vi "Get value by Variant.vi"(8 "error in (no error)":errorcluster, 11 "Numeric Column in":refnum<class "Numeric Column.lvclass">) -> (0 "error out":errorcluster, 2 "Variant":variant, 3 "Numeric Column out":refnum<class "Numeric Column.lvclass">)   [LabVIEW 2020, in "Basic Columns.lvlib" / "Numeric Column.lvclass"]
uses:
  Numeric Column.lvclass
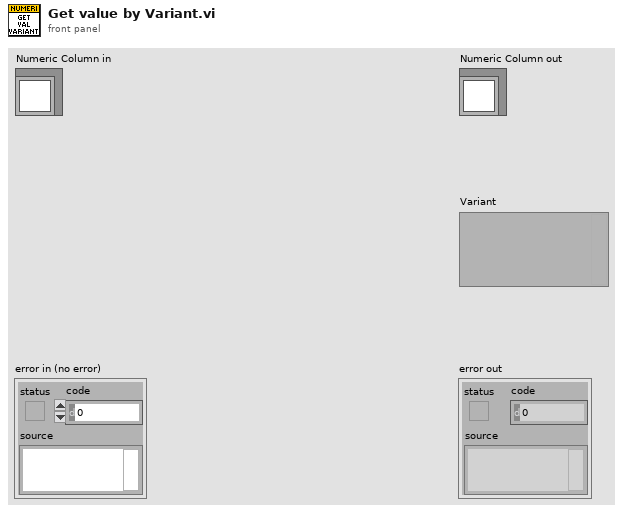
[diagram p1: front panel]
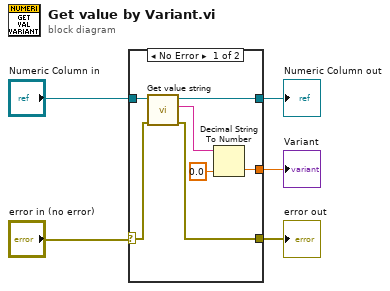
[diagram p0: block diagram]
diagram:
  n1 = case shown="No Error" "error in (no error)" {
    selector: "error in (no error)" -> [w10 w13]
    tunnel: "Numeric Column in" -> [w12 w14]
    tunnel: [w11 w14] -> w3
    tunnel: [w6 w13] -> w2
    tunnel: [w7 _] -> w1
    frame No Error {
      n2 = call-dynamic "Get value string.vi"("error in (no error)"=w10, "Column in"=w12) -> ("error out"=w6:errorcluster, "Value"=w9:string, "Column out"=w11:refnum<class "Numeric Column.lvclass">)  [unwired: 7 in]
      n3 = Decimal String To Number(string=w9, default (0L)=0.0) -> (number=w7:dbl)  [unwired: 1 in, 1 out]
    }
    frame Error {
    }
  }
  "error out" <- w2
  "Numeric Column out" <- w3
  "Variant" <- w1
